vi "FTW-TransferClient-UploadBegin.vi"(0 "Transfer Client":refnum<class "FTW-TransferClient-S3.lvclass">, 5 "Local Filepath":path, 7 "Remote Relative Filepath":string, 11 "error in":errorcluster) -> (4 "Transfer Client out":refnum<class "FTW-TransferClient-S3.lvclass">, 6 "Upload Events":refnum<event-registration>, 15 "error out":errorcluster)   [LabVIEW 2012, in "FTW-TransferClient-S3.lvclass"]
uses:
  FTW-TransferClient-S3.lvclass
  FTW-TransferClient-TransferProgress.ctl
  FTW-TransferClient-TransferStatus.ctl
  FTW-TransferClient-S3.lvclass/FTW-TransferClient-S3.ctl
  C:/Users/Jack/repo/ftw-master/Web/Transfer Client/S3/AWSSDK.dll
  AWSSDK.dll
  FTW-TransferClient-S3-ProcessUpload.vi
  FTW-TransferClient.lvclass
panel:
  # "Inputs"
  # "Outputs"
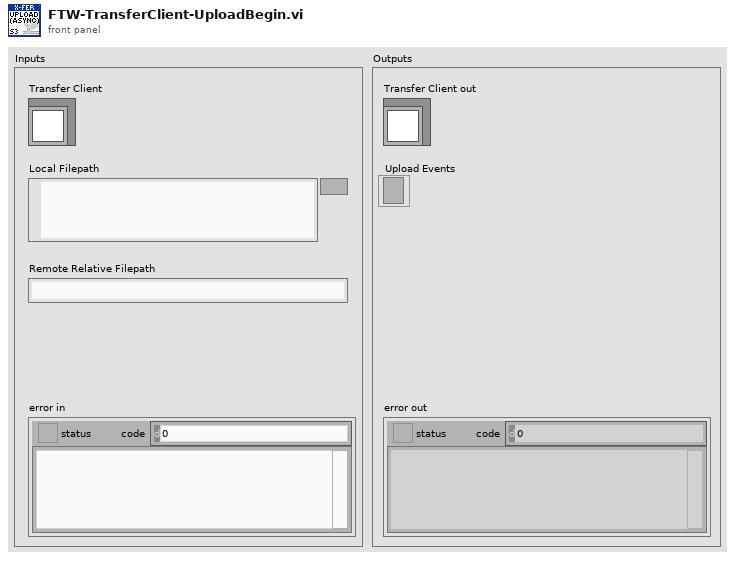
[diagram p1: front panel]
types:
  T1 = cluster{"Initial Timestamp":u32, "Transfer Progress":refnum<user-event>}
  T2 = typedef "FTW-Collection-KeyValuePair.ctl" = cluster{"Key":string, "Value":string}
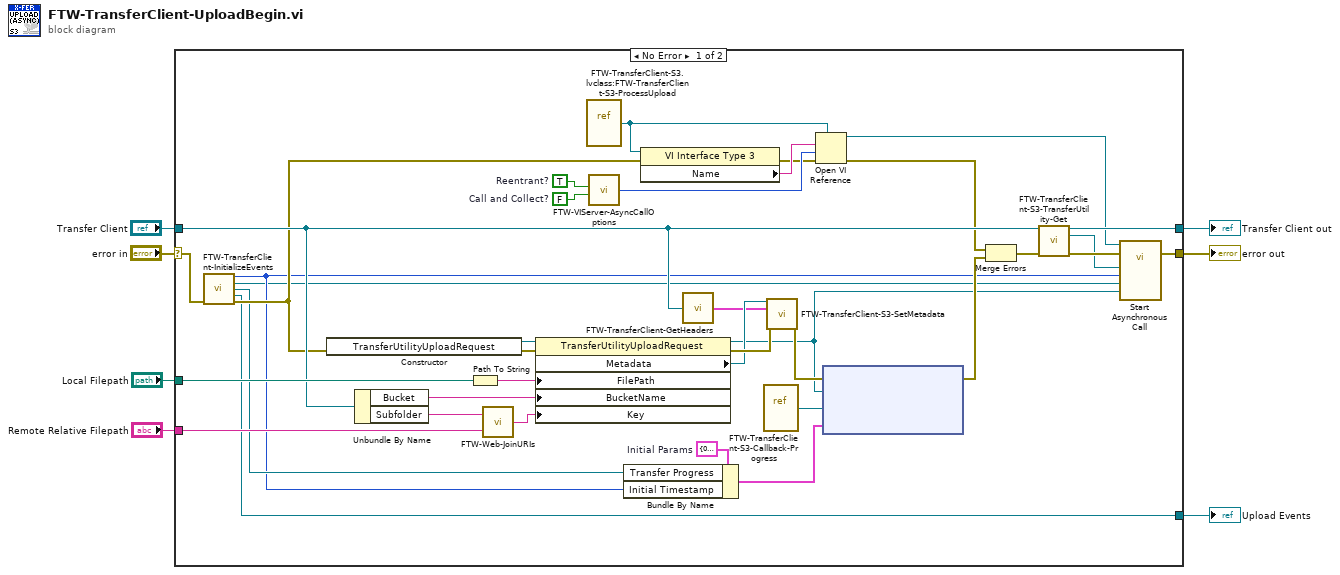
[diagram p0: block diagram]
diagram:
  n1 = case shown="No Error" "error in" {
    selector: "error in" -> [w16 w45]
    tunnel: "Local Filepath" -> [w42 _]
    tunnel: "Remote Relative Filepath" -> [w22 _]
    tunnel: [w29 w46] -> w5
    tunnel: [w27 w45] -> w4
    tunnel: "Transfer Client" -> [w26 w46]
    tunnel: [w13 _] -> w1
    frame No Error {
      w36 = T1 {"Initial Timestamp"=0, "Transfer Progress"=refnum}  # Initial Params
      w33 = FALSE  # Call and Collect?
      w32 = TRUE  # Reentrant?
      n2 = call "FTW-TransferClient-InitializeEvents.vi"("error in"=w16) -> ("Transfer Begin Timestamp"=w12:u32, "Transfer Complete"=w9:refnum<user-event>, "Transfer Progress"=w14:refnum<user-event>, "Transfer Events"=w13:refnum<event-registration>, "error out"=w15:errorcluster)  [unwired: 10 in]
      n3 = constructor class="TransferUtilityUploadRequest"(error in=w15) -> (reference out=w43:refnum<k24>, error out=w44:errorcluster)  [unwired: 2 in, 1 out]
      n4 = Unbundle By Name(w26) -> ("Bucket"=w41:string, "Subfolder"=w21:string)
      n5 = Path To String(path=w42) -> (string=w19:string)
      n6 = call "FTW-Web-JoinURIs.vi"("Base URI"=w21, "Relative URI"=w22) -> ("Output"=w20:string)  [unwired: 3 in]
      n7 = property class="TransferUtilityUploadRequest"(reference=w43, error in=w44, "FilePath"=w19, "BucketName"=w41, "Key"=w20) -> (reference out=w8:refnum<k24>, error out=w40:errorcluster, "Metadata"=w38:refnum<k24>)
      n8 = vi-ref "FTW-TransferClient-S3.lvclass:FTW-TransferClient-S3-ProcessUpload.vi"() -> (w17:refnum<vi>)
      n9 = call "FTW-VIServer-AsyncCallOptions.vi"("Call and Collect?"=w33, "Reentrant?"=w32) -> ("Open VI Ref Options"=w34:i32)  [unwired: 4 in]
      n10 = Bundle By Name(cluster=w36, "Transfer Progress"=w14, "Initial Timestamp"=w12) -> (w35:T1)
      n11 = property class="VI Interface Type 3"(reference=w17, error in=w15) -> (error out=w30:errorcluster, "Name"=w31:string)  [unwired: 1 out]
      n12 = call "FTW-TransferClient-GetHeaders.vi"("Transfer Client"=w26) -> ("Headers"=w37:T2[])
      n13 = vi-ref "FTW-TransferClient-S3-Callback-Progress.vi"() -> ("vi reference"=w18:refnum<vi>)
      n14 = call "FTW-TransferClient-S3-SetMetadata.vi"("Metadata"=w38, "Metadata Collection"=w37, "error in"=w40) -> ("error out"=w39:errorcluster)  [unwired: 12 in]
      n15 = Open VI Reference(type specifier VI Refnum (for type only)=w17, vi path=w31, options=w34, error in (no error)=w30) -> (vi reference=w10:refnum<vi>, error out=w25:errorcluster)  [unwired: 2 in]
      n16 = node(w39, w8, w18, w35) -> (w28:errorcluster)  [unwired: 1 in, 1 out]
      n17 = Merge Errors(w25, w28) -> (w23:errorcluster)
      n18 = call "FTW-TransferClient-S3-TransferUtility-Get.vi"("Transfer Client"=w26, "error in"=w23) -> ("Transfer Client out"=w29:refnum<class "FTW-TransferClient-S3.lvclass">, "Transfer Utility ref"=w11:refnum<k24>, "error out"=w24:errorcluster)  [unwired: 11 in]
      n19 = call-by-ref "Start Asynchronous Call"(reference=w10, error in=w24, "Upload Request"=w8, "Transfer Status"=w9, "Initial Time"=w12, "Transfer Utility"=w11) -> (error out=w27:errorcluster)  [unwired: 8 in, 1 out]
    }
    frame Error {
    }
  }
  "error out" <- w4
  "Transfer Client out" <- w5
  "Upload Events" <- w1
